vi "RNP.vi"(0 "System no.":i32=1 min=1 max=4 step=1, 2 "PiezoWalkChannel":string[](array[string]), 3 "Adj. voltage":dbl[](array[numeric]) format="%.6f", 4 "No.of digits":i16=4, 5 "error in":errorcluster, 12 "Stop refnum":refnum<vi>) -> (19 "error out":errorcluster)   [LabVIEW 2020]
doc: "Relax piezos of given PiezoWalk® channels without motion and wait until procedure has stopped. The aim of this procedure is to reduce all applied voltages when the target is reached and thus to increase the lifetime of the piezos. To compensate a preload which would lead to a small motion of the slider when the piezo voltage is zero an adjustment voltage can be applied. VI will also stop if Stop refnum or Local stop is TRUE. \n\nE-712: Adj. voltage must be zero to set the voltages to 0. Servo must be disabled for the axis to which the PiezoWalk channel is assigned (open-loop operation). RNP starts the simple relax procedure. To start the iterative relax procedure which is available for axes driven by one PiezoWalk® drive and measured by one sensor only, use SVO.vi to switch servo off for these axes. In nanostepping mode, RNP must be used in the following cases due to the possibility to perform parts of complete steps:\nAfter stepping motion in open-loop operation a relax procedure is required before analog mode motion is possible\nSwitching to closed-loop operation (set servo on with SVO) is only possible after a relax procedure. \n\nE-755: The RNP procedure is automatically performed when the servo is switched off and when RTO is used.\n\nE-861: Adj. voltage must be zero to set the voltages to 0.\nServo must be disabled for the commanded axis prior to using this command (open-loop operation).\nIn open-loop operation, an RNP command must be sent each time the motion mode is to be changed from stepping motion (OSM, OMA, OMR) to analog motion (OAD) or vice versa.\nAfter open-loop analog motion was done with OAD, an RNP command must be sent before the servo can be switched on with SVO for closed-loop operation.\nThe RNP procedure can take up to four times the slewrate value (parameter ID 0x7000002; can be changed with SPA and SEP).\nYou can query the current state of the system (E-861 and NEXACT® linear drive) using #4 and SRG?."
panel:
  in  "Local stop":bool
  # "Relax piezos of given PiezoWalk® channels without motion and\nwaits until procedure has stopped. VI will also stop\nif Stop refnum or Local stop is TRUE."
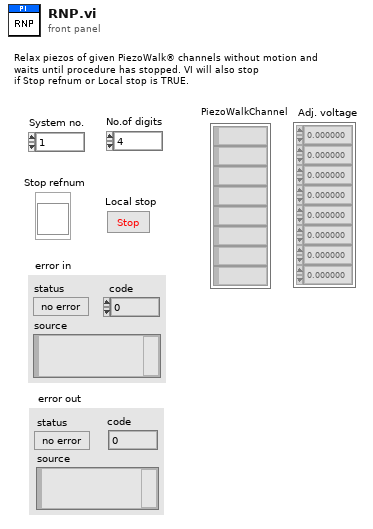
[diagram p1: front panel]
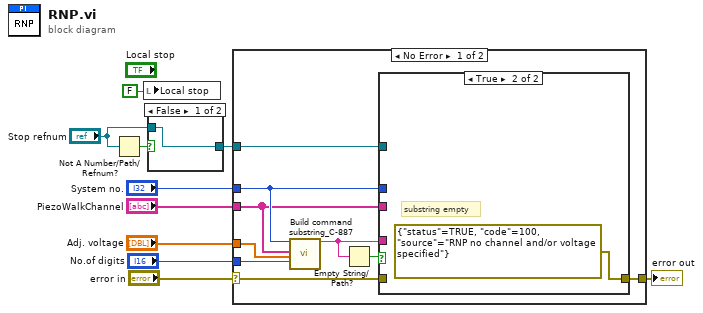
[diagram p0: block diagram]
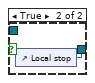
[diagram p2: hidden frame]
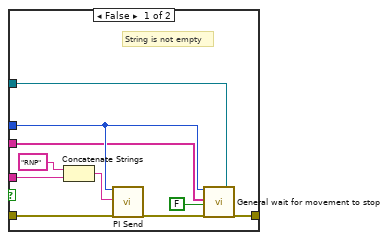
[diagram p3: hidden frame]
diagram:
  n1 = Not A Number/Path/Refnum?(number/path/refnum="Stop refnum") -> (NaN/Path/Refnum?=w4:bool)
  n2 = local write "Local stop"(FALSE ("Local stop")) -> ()
  n3 = case shown="False" w4 {
    tunnel: [w11 w12] -> w2
    tunnel: "Stop refnum" -> [w11 _]
    frame False {
    }
    frame True {
      n4 = control-ref of="Local stop"() -> (w12:refnum<vi>)
    }
  }
  n5 = case shown="No Error" "error in" {
    selector: "error in" -> [w15 w33]
    tunnel: [w21 w33] -> w10
    tunnel: "Adj. voltage" -> [w20 _]
    tunnel: "No.of digits" -> [w19 _]
    tunnel: "System no." -> [w18 _]
    tunnel: "PiezoWalkChannel" -> [w17 _]
    tunnel: w2 -> [w16 _]
    frame No Error {
      n6 = call "Build command substring_C-887.vi"("System no."=w18, "Affected axes"=w17, "Parameters"=w20, "No. of digits"=w19) -> ("Command substring"=w13:string)  [unwired: 3 in, 12 out]
      n7 = Empty String/Path?(string/path=w13) -> (empty?=w14:bool)
      n8 = case shown="True" w14 {
        tunnel: w13 -> [w30 _]
        tunnel: [w26 errorcluster {"status"=TRUE, "code"=100, "source"="RNP no channel and/or voltage specified"} ("error out")] -> w21
        tunnel: w15 -> [w28 _]
        tunnel: w18 -> [w25 _]
        tunnel: w17 -> [w23 _]
        tunnel: w16 -> [w22 _]
        frame False {
          # "String is not empty"
          n9 = Concatenate Strings("RNP", w30) -> (w29:string)
          n10 = call "PI Send.vi"("System no."=w25, "String to send"=w29, "error in"=w28) -> ("error out"=w27:errorcluster)  [unwired: 3 in, 13 out]
          n11 = call "General wait for movement to stop.vi"("System no."=w25, "Axes to wait for"=w23, "All axes?"=FALSE, "error in"=w27, "Stop refnum"=w22) -> ("error out"=w26:errorcluster)  [unwired: 3 in, 11 out]
        }
        frame True {
          # "substring empty"
        }
      }
    }
    frame Error {
    }
  }
  "error out" <- w10
